vi "Get Field Units.vi"(2 "error in":T2, 3 "Z-Axis Communications Config":T1={"GPIB address"=22, "GPIB bus"=0, "connection ID"=refnum, "IP"="111.111.111.1", "Active Comm Interface"=0, "Serial Port"="", "Programmer Type"=0} {"Active Comm Interface" items=["TCP/IP (Model 430 Only)", "RS232", "IEEE488"]; "Programmer Type" items=["Model 430", "Model 420"]}) -> (0 "error out":T2, 1 "Field Units":enum16{"kg", "t"}(ring))   [LabVIEW 2018]
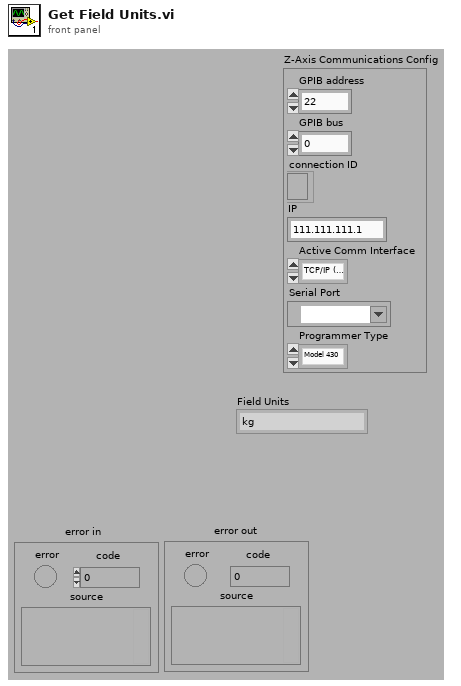
[diagram p1: front panel]
types:
  T1 = cluster{"GPIB address":i16, "GPIB bus":i16, "connection ID":refnum<k5>, "IP":string, "Active Comm Interface":u16, "Serial Port":refnum<visa-resource-name>, "Programmer Type":u16}
  T2 = cluster{"error":bool, "code":i32, "source":string}
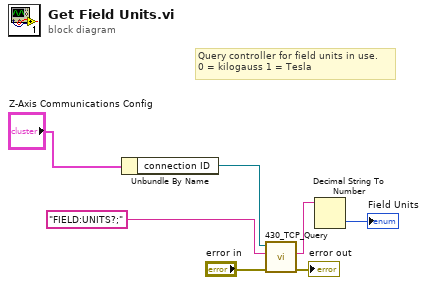
[diagram p0: block diagram]
diagram:
  # "Query controller for field units in use.\n0 = kilogauss 1 = Tesla"
  n1 = Unbundle By Name("Z-Axis Communications Config") -> ("connection ID"=w1:refnum<k5>)
  n2 = call "430_TCP_Query.vi"("error in (no error)"="error in", "Command"="FIELD:UNITS?;" ("Input query"), "connection ID"=w1) -> ("error out"=→"error out":errorcluster, "Response"=w4:string)  [unwired: 4 in, 3 out]
  n3 = Decimal String To Number(string=w4) -> (number=→"Field Units":i32)  [unwired: 2 in, 1 out]
